vi "HAND_AUTO.vi"() -> ()   [LabVIEW 2014]
uses:
  <vilib>/Platform/TimedLoop/XDataNode/timing_clust.ctl
  <vilib>/Platform/TimedLoop/XDataNode/nitl_modes.ctl
  <vilib>/Platform/TimedLoop/XDataNode/wakeup.ctl
  <vilib>/platform/TimedLoop/XDataNode/XDataNode.xnode
  <vilib>/Platform/TimedLoop/XDataNode/XDNodeRunTimeDep.lvlib
panel:
  out "EMERGENCY":bool
  out "TIME":bool
  out "HAND/AUTO":bool
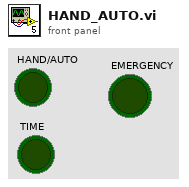
[diagram p1: front panel]
types:
  T1 = typedef "XDNodeRunTimeDep.lvlib/timing_clust.ctl" = cluster{"Expected End [f-1]":u64, "Actual End [f-1]":u64, "Finished Late? [f-1]":bool, "Expected End [i-1]":u64, "Actual End [i-1]":u64, "Finished Late? [i-1]":bool, "Expected Start [i]":u64, "Actual Start [i]":u64, "Expected Start [f]":u64, "Actual Start [f]":u64, "Source Name":string, "Structure Name":string, "Period":i64, "Deadline":i64, "Offset":i64, "Start":i64, "Priority":i32, "Timeout":i32, "Mode":T2, "Wakeup Reason":T3, "Error":errorcluster, "Source Type":string, "Secondary Source Type":string, "Global End Time":u64, "Global Start Time":u64, "Frame Duration":u64, "Iteration Duration":u64, "Assigned CPU":i32, "I/O Scan Engine Mode":u32}
  T2 = typedef "XDNodeRunTimeDep.lvlib/nitl_modes.ctl" = enum32{"No Change", "Process missed periods, maintain original phase", "Discard missed periods, maintain original phase", "Process missed periods, ignore original phase", "Discard missed periods, ignore original phase"}
  T3 = typedef "XDNodeRunTimeDep.lvlib/wakeup.ctl" = enum32{"Normal", "Aborted", "Asynchronous wakeup", "Timing source error", "Timed loop error", "Timeout"}
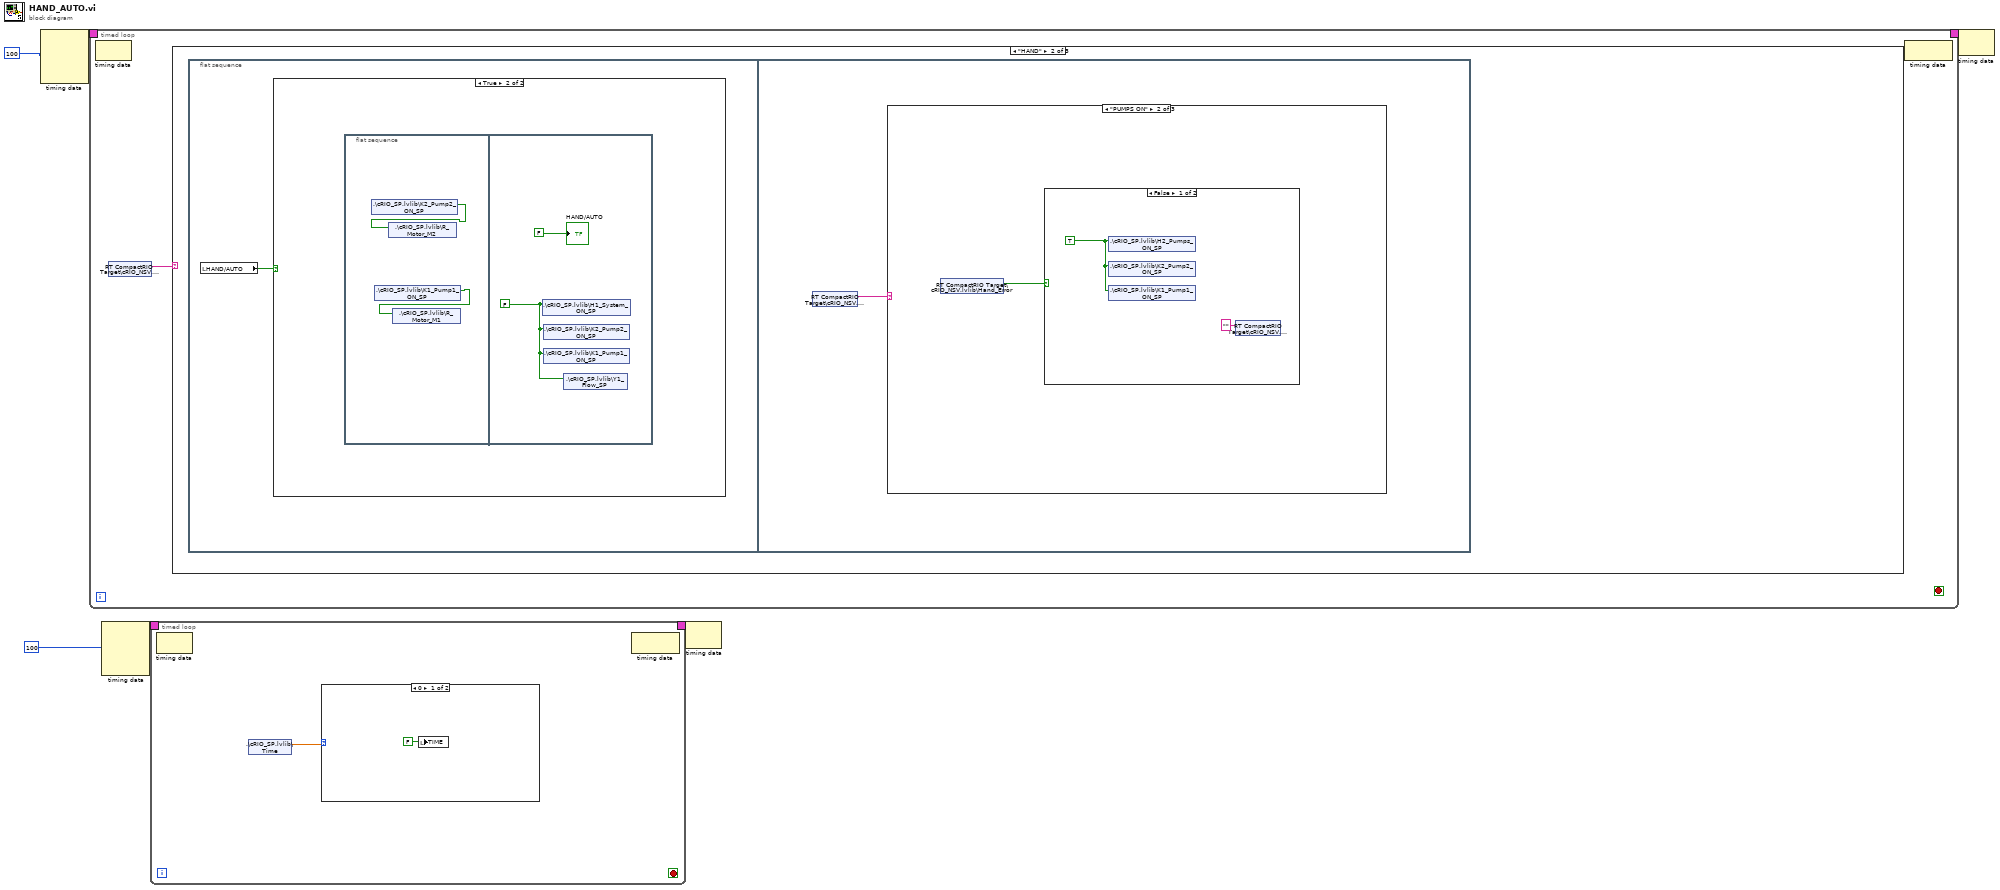
[diagram p0: block diagram]
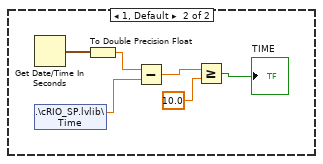
[diagram p2: hidden frame]
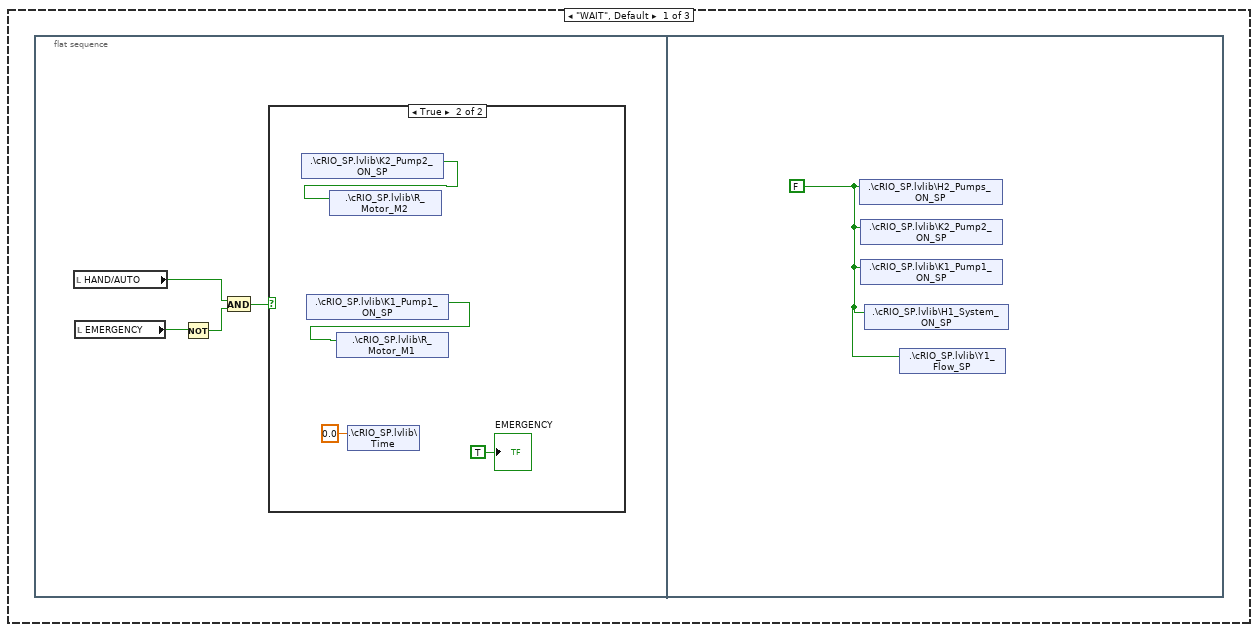
[diagram p3: hidden frame]
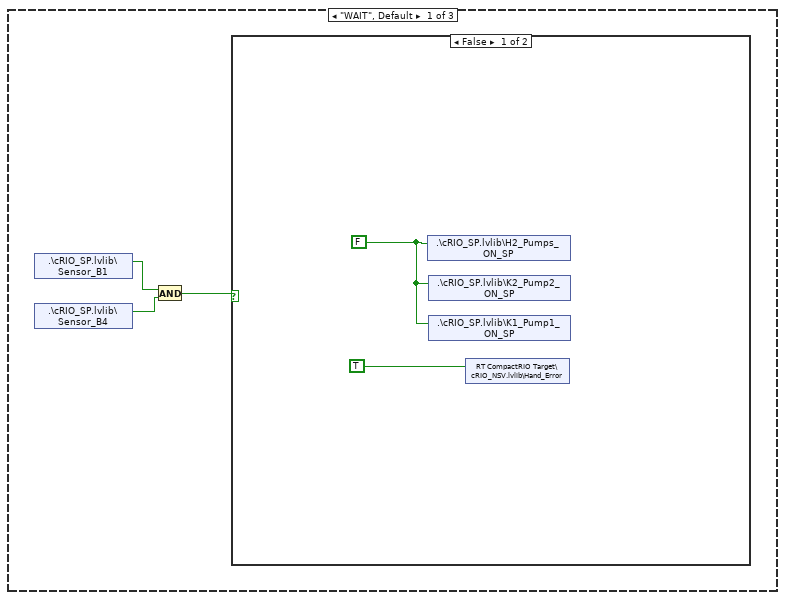
[diagram p6: hidden frame]
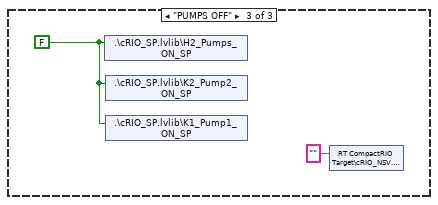
[diagram p9: hidden frame]
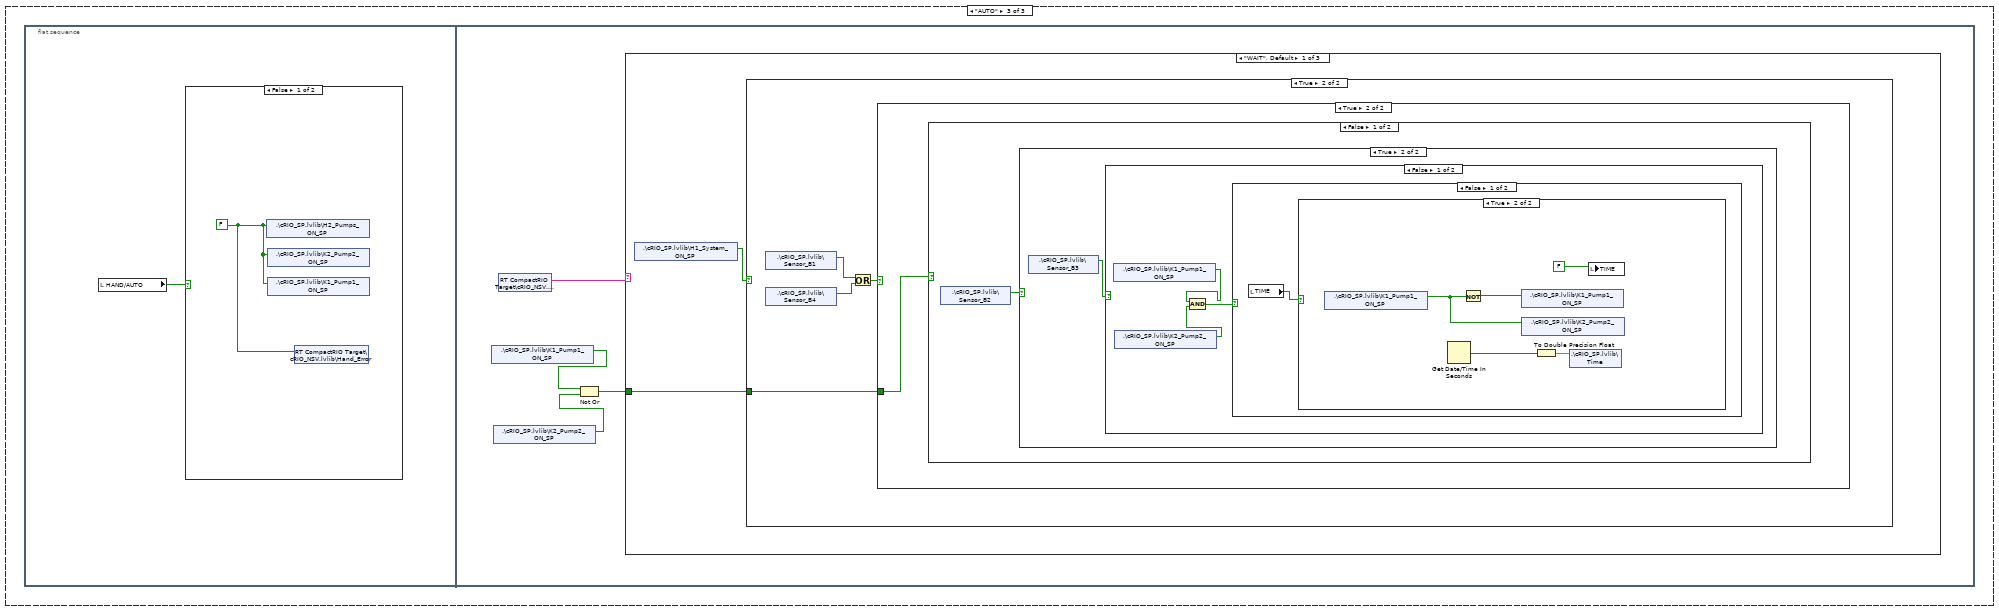
[diagram p10: hidden frame]
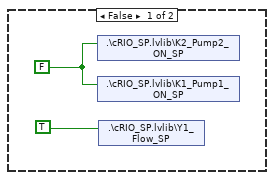
[diagram p13: hidden frame]
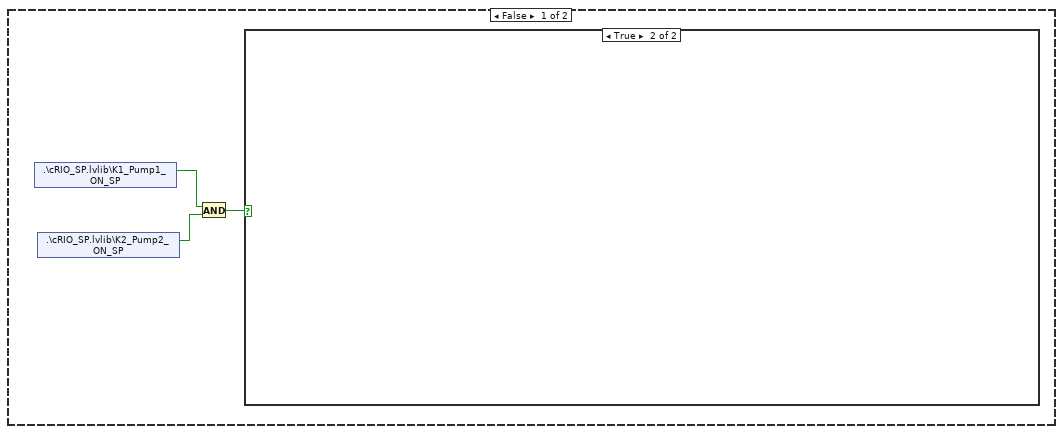
[diagram p14: hidden frame]
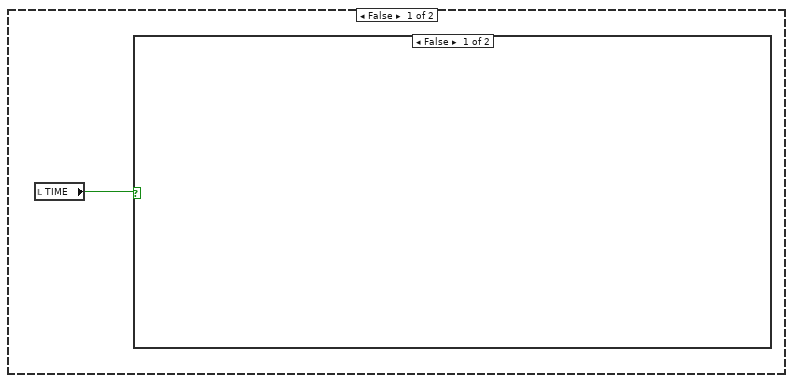
[diagram p15: hidden frame]
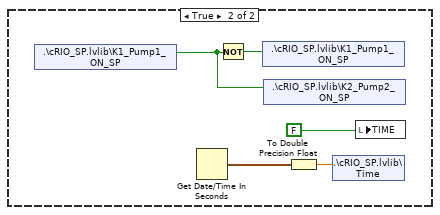
[diagram p16: hidden frame]
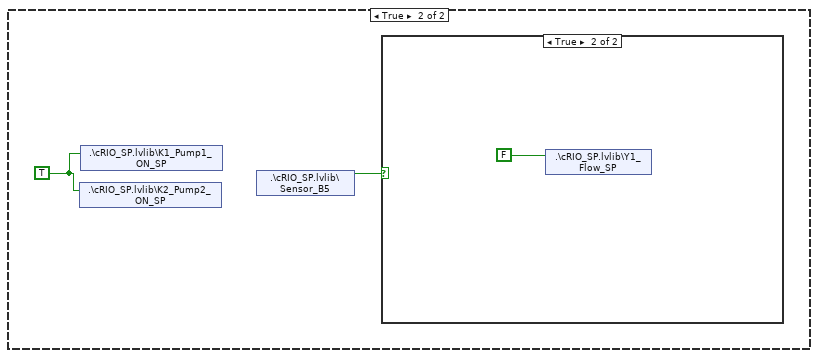
[diagram p19: hidden frame]
diagram:
  n1 = node-c288(i64 100 ("Period")) -> (w6:T1)  [unwired: 3 in]
  n2 = timed-loop {
    timing: w6 -> [_]
    timing-out: [_] -> w5
    stop <- _ stop-if-true
    n3 = node-c288() -> ()  [unwired: 1 in, 1 out]
    n4 = shared-variable "RT CompactRIO Target\\cRIO_NSV.lvlib\\State"() -> (w7:string)  [unwired: 1 in, 1 out]
    n5 = case shown="\"HAND\"" w7 {
      frame "WAIT", Default {
        n6 = flat-sequence {
          frame #0 {
            n7 = local read "HAND/AUTO"() -> (w10:bool)
            n8 = local read "EMERGENCY"() -> (w12:bool)
            n9 = Not(x=w12) -> (.not. x?=w11:bool)
            n10 = And(x=w10, y=w11) -> (x .and. y?=w13:bool)
            n11 = case shown="True" w13 {
              frame False {
              }
              frame True {
                n12 = shared-variable ".\\cRIO_SP.lvlib\\K2_Pump2_ON_SP"() -> (w17:bool)  [unwired: 1 in, 1 out]
                n13 = shared-variable ".\\cRIO_SP.lvlib\\K1_Pump1_ON_SP"() -> (w16:bool)  [unwired: 1 in, 1 out]
                n14 = shared-variable ".\\cRIO_SP.lvlib\\R_Motor_M2"(w17) -> ()  [unwired: 1 in, 1 out]
                n15 = shared-variable ".\\cRIO_SP.lvlib\\R_Motor_M1"(w16) -> ()  [unwired: 1 in, 1 out]
                n16 = shared-variable ".\\cRIO_SP.lvlib\\Time"(0.0 ("Time")) -> ()  [unwired: 1 in, 1 out]
                "EMERGENCY" <- TRUE ("EMERGENCY")
              }
            }
          }
          frame #1 {
            w18 = FALSE
            n17 = shared-variable ".\\cRIO_SP.lvlib\\H2_Pumps_ON_SP"(w18) -> ()  [unwired: 1 in, 1 out]
            n18 = shared-variable ".\\cRIO_SP.lvlib\\K2_Pump2_ON_SP"(w18) -> ()  [unwired: 1 in, 1 out]
            n19 = shared-variable ".\\cRIO_SP.lvlib\\K1_Pump1_ON_SP"(w18) -> ()  [unwired: 1 in, 1 out]
            n20 = shared-variable ".\\cRIO_SP.lvlib\\H1_System_ON_SP"(w18) -> ()  [unwired: 1 in, 1 out]
            n21 = shared-variable ".\\cRIO_SP.lvlib\\Y1_Flow_SP"(w18) -> ()  [unwired: 1 in, 1 out]
          }
        }
      }
      frame "HAND" {
        n22 = flat-sequence {
          frame #0 {
            n23 = local read "HAND/AUTO"() -> (w19:bool)
            n24 = case shown="True" w19 {
              frame False {
              }
              frame True {
                n25 = flat-sequence {
                  frame #0 {
                    n26 = shared-variable ".\\cRIO_SP.lvlib\\K2_Pump2_ON_SP"() -> (w20:bool)  [unwired: 1 in, 1 out]
                    n27 = shared-variable ".\\cRIO_SP.lvlib\\K1_Pump1_ON_SP"() -> (w21:bool)  [unwired: 1 in, 1 out]
                    n28 = shared-variable ".\\cRIO_SP.lvlib\\R_Motor_M2"(w20) -> ()  [unwired: 1 in, 1 out]
                    n29 = shared-variable ".\\cRIO_SP.lvlib\\R_Motor_M1"(w21) -> ()  [unwired: 1 in, 1 out]
                  }
                  frame #1 {
                    w23 = FALSE
                    n30 = shared-variable ".\\cRIO_SP.lvlib\\H1_System_ON_SP"(w23) -> ()  [unwired: 1 in, 1 out]
                    n31 = shared-variable ".\\cRIO_SP.lvlib\\K2_Pump2_ON_SP"(w23) -> ()  [unwired: 1 in, 1 out]
                    n32 = shared-variable ".\\cRIO_SP.lvlib\\K1_Pump1_ON_SP"(w23) -> ()  [unwired: 1 in, 1 out]
                    n33 = shared-variable ".\\cRIO_SP.lvlib\\Y1_Flow_SP"(w23) -> ()  [unwired: 1 in, 1 out]
                    "HAND/AUTO" <- FALSE
                  }
                }
              }
            }
          }
          frame #1 {
            n34 = shared-variable "RT CompactRIO Target\\cRIO_NSV.lvlib\\Tasks"() -> (w24:string)  [unwired: 1 in, 1 out]
            n35 = case shown="\"PUMPS ON\"" w24 {
              frame "WAIT", Default {
                n36 = shared-variable ".\\cRIO_SP.lvlib\\Sensor_B1"() -> (w26:bool)  [unwired: 1 in, 1 out]
                n37 = shared-variable ".\\cRIO_SP.lvlib\\Sensor_B4"() -> (w27:bool)  [unwired: 1 in, 1 out]
                n38 = And(x=w26, y=w27) -> (x .and. y?=w25:bool)
                n39 = case shown="False" w25 {
                  frame False {
                    w29 = FALSE
                    n40 = shared-variable ".\\cRIO_SP.lvlib\\H2_Pumps_ON_SP"(w29) -> ()  [unwired: 1 in, 1 out]
                    n41 = shared-variable ".\\cRIO_SP.lvlib\\K2_Pump2_ON_SP"(w29) -> ()  [unwired: 1 in, 1 out]
                    n42 = shared-variable ".\\cRIO_SP.lvlib\\K1_Pump1_ON_SP"(w29) -> ()  [unwired: 1 in, 1 out]
                    n43 = shared-variable "RT CompactRIO Target\\cRIO_NSV.lvlib\\Hand_Error"(TRUE) -> ()  [unwired: 1 in, 1 out]
                  }
                  frame True {
                  }
                }
              }
              frame "PUMPS ON" {
                n44 = shared-variable "RT CompactRIO Target\\cRIO_NSV.lvlib\\Hand_Error"() -> (w30:bool)  [unwired: 1 in, 1 out]
                n45 = case shown="False" w30 {
                  frame False {
                    w32 = TRUE
                    n46 = shared-variable ".\\cRIO_SP.lvlib\\H2_Pumps_ON_SP"(w32) -> ()  [unwired: 1 in, 1 out]
                    n47 = shared-variable ".\\cRIO_SP.lvlib\\K2_Pump2_ON_SP"(w32) -> ()  [unwired: 1 in, 1 out]
                    n48 = shared-variable ".\\cRIO_SP.lvlib\\K1_Pump1_ON_SP"(w32) -> ()  [unwired: 1 in, 1 out]
                    n49 = shared-variable "RT CompactRIO Target\\cRIO_NSV.lvlib\\Tasks"("" ("Tasks")) -> ()  [unwired: 1 in, 1 out]
                  }
                  frame True {
                  }
                }
              }
              frame "PUMPS OFF" {
                w34 = FALSE
                n50 = shared-variable ".\\cRIO_SP.lvlib\\H2_Pumps_ON_SP"(w34) -> ()  [unwired: 1 in, 1 out]
                n51 = shared-variable ".\\cRIO_SP.lvlib\\K2_Pump2_ON_SP"(w34) -> ()  [unwired: 1 in, 1 out]
                n52 = shared-variable ".\\cRIO_SP.lvlib\\K1_Pump1_ON_SP"(w34) -> ()  [unwired: 1 in, 1 out]
                n53 = shared-variable "RT CompactRIO Target\\cRIO_NSV.lvlib\\Tasks"("" ("Tasks")) -> ()  [unwired: 1 in, 1 out]
              }
            }
          }
        }
      }
      frame "AUTO" {
        n54 = flat-sequence {
          frame #0 {
            n55 = local read "HAND/AUTO"() -> (w35:bool)
            n56 = case shown="False" w35 {
              frame False {
                w36 = FALSE
                n57 = shared-variable ".\\cRIO_SP.lvlib\\H2_Pumps_ON_SP"(w36) -> ()  [unwired: 1 in, 1 out]
                n58 = shared-variable ".\\cRIO_SP.lvlib\\K2_Pump2_ON_SP"(w36) -> ()  [unwired: 1 in, 1 out]
                n59 = shared-variable ".\\cRIO_SP.lvlib\\K1_Pump1_ON_SP"(w36) -> ()  [unwired: 1 in, 1 out]
                n60 = shared-variable "RT CompactRIO Target\\cRIO_NSV.lvlib\\Hand_Error"(w36) -> ()  [unwired: 1 in, 1 out]
              }
              frame True {
              }
            }
          }
          frame #1 {
            n61 = shared-variable ".\\cRIO_SP.lvlib\\K1_Pump1_ON_SP"() -> (w38:bool)  [unwired: 1 in, 1 out]
            n62 = shared-variable ".\\cRIO_SP.lvlib\\K2_Pump2_ON_SP"() -> (w37:bool)  [unwired: 1 in, 1 out]
            n63 = shared-variable "RT CompactRIO Target\\cRIO_NSV.lvlib\\Tasks"() -> (w40:string)  [unwired: 1 in, 1 out]
            n64 = Not Or(1:w37, 2:w38) -> (0:w39:bool)
            n65 = case shown="\"WAIT\", Default" w40 {
              tunnel: w39 -> [w41 _ _]
              frame "WAIT", Default {
                n66 = shared-variable ".\\cRIO_SP.lvlib\\H1_System_ON_SP"() -> (w42:bool)  [unwired: 1 in, 1 out]
                n67 = case shown="True" w42 {
                  tunnel: w41 -> [_ w44]
                  frame False {
                  }
                  frame True {
                    n68 = shared-variable ".\\cRIO_SP.lvlib\\Sensor_B1"() -> (w43:bool)  [unwired: 1 in, 1 out]
                    n69 = shared-variable ".\\cRIO_SP.lvlib\\Sensor_B4"() -> (w45:bool)  [unwired: 1 in, 1 out]
                    n70 = Or(x=w43, y=w45) -> (x .or. y?=w46:bool)
                    n71 = case shown="True" w46 {
                      tunnel: w44 -> [_ w49]
                      frame False {
                        w48 = FALSE
                        n72 = shared-variable ".\\cRIO_SP.lvlib\\K2_Pump2_ON_SP"(w48) -> ()  [unwired: 1 in, 1 out]
                        n73 = shared-variable ".\\cRIO_SP.lvlib\\K1_Pump1_ON_SP"(w48) -> ()  [unwired: 1 in, 1 out]
                        n74 = shared-variable ".\\cRIO_SP.lvlib\\Y1_Flow_SP"(TRUE) -> ()  [unwired: 1 in, 1 out]
                      }
                      frame True {
                        n75 = case shown="False" w49 {
                          frame False {
                            n76 = shared-variable ".\\cRIO_SP.lvlib\\Sensor_B2"() -> (w50:bool)  [unwired: 1 in, 1 out]
                            n77 = case shown="True" w50 {
                              frame False {
                                n78 = shared-variable ".\\cRIO_SP.lvlib\\K1_Pump1_ON_SP"() -> (w51:bool)  [unwired: 1 in, 1 out]
                                n79 = shared-variable ".\\cRIO_SP.lvlib\\K2_Pump2_ON_SP"() -> (w52:bool)  [unwired: 1 in, 1 out]
                                n80 = And(x=w51, y=w52) -> (x .and. y?=w53:bool)
                                n81 = case shown="True" w53 {
                                frame False {
                                n82 = local read "TIME"() -> (w54:bool)
                                n83 = case shown="False" w54 {
                                frame False {
                                }
                                frame True {
                                n84 = shared-variable ".\\cRIO_SP.lvlib\\K1_Pump1_ON_SP"() -> (w58:bool)  [unwired: 1 in, 1 out]
                                n85 = Get Date/Time In Seconds() -> (seconds since 1Jan1904=w55:timestamp)
                                n86 = Not(x=w58) -> (.not. x?=w59:bool)
                                n87 = shared-variable ".\\cRIO_SP.lvlib\\K1_Pump1_ON_SP"(w59) -> ()  [unwired: 1 in, 1 out]
                                n88 = shared-variable ".\\cRIO_SP.lvlib\\K2_Pump2_ON_SP"(w58) -> ()  [unwired: 1 in, 1 out]
                                n89 = To Double Precision Float(number=w55) -> (double precision float=w56:dbl)
                                n90 = shared-variable ".\\cRIO_SP.lvlib\\Time"(w56) -> ()  [unwired: 1 in, 1 out]
                                n91 = local write "TIME"(FALSE) -> ()
                                }
                                }
                                }
                                frame True {
                                }
                                }
                              }
                              frame True {
                                n92 = shared-variable ".\\cRIO_SP.lvlib\\Sensor_B3"() -> (w60:bool)  [unwired: 1 in, 1 out]
                                n93 = case shown="False" w60 {
                                frame False {
                                n94 = shared-variable ".\\cRIO_SP.lvlib\\K1_Pump1_ON_SP"() -> (w62:bool)  [unwired: 1 in, 1 out]
                                n95 = shared-variable ".\\cRIO_SP.lvlib\\K2_Pump2_ON_SP"() -> (w61:bool)  [unwired: 1 in, 1 out]
                                n96 = And(x=w62, y=w61) -> (x .and. y?=w63:bool)
                                n97 = case shown="False" w63 {
                                frame False {
                                n98 = local read "TIME"() -> (w64:bool)
                                n99 = case shown="True" w64 {
                                frame False {
                                }
                                frame True {
                                n100 = shared-variable ".\\cRIO_SP.lvlib\\K1_Pump1_ON_SP"() -> (w68:bool)  [unwired: 1 in, 1 out]
                                n101 = Get Date/Time In Seconds() -> (seconds since 1Jan1904=w65:timestamp)
                                n102 = Not(x=w68) -> (.not. x?=w69:bool)
                                n103 = shared-variable ".\\cRIO_SP.lvlib\\K1_Pump1_ON_SP"(w69) -> ()  [unwired: 1 in, 1 out]
                                n104 = shared-variable ".\\cRIO_SP.lvlib\\K2_Pump2_ON_SP"(w68) -> ()  [unwired: 1 in, 1 out]
                                n105 = To Double Precision Float(number=w65) -> (double precision float=w66:dbl)
                                n106 = shared-variable ".\\cRIO_SP.lvlib\\Time"(w66) -> ()  [unwired: 1 in, 1 out]
                                n107 = local write "TIME"(FALSE) -> ()
                                }
                                }
                                }
                                frame True {
                                }
                                }
                                }
                                frame True {
                                w71 = TRUE
                                n108 = shared-variable ".\\cRIO_SP.lvlib\\K2_Pump2_ON_SP"(w71) -> ()  [unwired: 1 in, 1 out]
                                n109 = shared-variable ".\\cRIO_SP.lvlib\\K1_Pump1_ON_SP"(w71) -> ()  [unwired: 1 in, 1 out]
                                n110 = shared-variable ".\\cRIO_SP.lvlib\\Sensor_B5"() -> (w70:bool)  [unwired: 1 in, 1 out]
                                n111 = case shown="True" w70 {
                                frame False {
                                }
                                frame True {
                                n112 = shared-variable ".\\cRIO_SP.lvlib\\Y1_Flow_SP"(FALSE) -> ()  [unwired: 1 in, 1 out]
                                }
                                }
                                }
                                }
                              }
                            }
                          }
                          frame True {
                            n113 = shared-variable ".\\cRIO_SP.lvlib\\Sensor_B2"() -> (w73:bool)  [unwired: 1 in, 1 out]
                            n114 = case shown="True" w73 {
                              frame False {
                              }
                              frame True {
                                n115 = Get Date/Time In Seconds() -> (seconds since 1Jan1904=w74:timestamp)
                                n116 = shared-variable ".\\cRIO_SP.lvlib\\K1_Pump1_ON_SP"(TRUE) -> ()  [unwired: 1 in, 1 out]
                                n117 = To Double Precision Float(number=w74) -> (double precision float=w75:dbl)
                                n118 = shared-variable ".\\cRIO_SP.lvlib\\Time"(w75) -> ()  [unwired: 1 in, 1 out]
                              }
                            }
                          }
                        }
                      }
                    }
                  }
                }
              }
              frame "SYSTEM ON" {
                w80 = TRUE
                n119 = shared-variable ".\\cRIO_SP.lvlib\\R_Motor_M1"() -> (w78:bool)  [unwired: 1 in, 1 out]
                n120 = shared-variable ".\\cRIO_SP.lvlib\\R_Motor_M2"() -> (w77:bool)  [unwired: 1 in, 1 out]
                n121 = shared-variable ".\\cRIO_SP.lvlib\\Y1_Flow_SP"(w80) -> ()  [unwired: 1 in, 1 out]
                n122 = shared-variable ".\\cRIO_SP.lvlib\\H1_System_ON_SP"(w80) -> ()  [unwired: 1 in, 1 out]
                n123 = shared-variable ".\\cRIO_SP.lvlib\\K1_Pump1_ON_SP"(w78) -> ()  [unwired: 1 in, 1 out]
                n124 = shared-variable ".\\cRIO_SP.lvlib\\K2_Pump2_ON_SP"(w77) -> ()  [unwired: 1 in, 1 out]
                n125 = shared-variable "RT CompactRIO Target\\cRIO_NSV.lvlib\\Tasks"("" ("Tasks")) -> ()  [unwired: 1 in, 1 out]
              }
              frame "SYSTEM OFF" {
                n126 = flat-sequence {
                  frame #0 {
                    n127 = local read "HAND/AUTO"() -> (w82:bool)
                    n128 = local read "EMERGENCY"() -> (w84:bool)
                    n129 = Not(x=w84) -> (.not. x?=w81:bool)
                    n130 = And(x=w82, y=w81) -> (x .and. y?=w83:bool)
                    n131 = case shown="True" w83 {
                      frame False {
                        n132 = Get Date/Time In Seconds() -> (seconds since 1Jan1904=w85:timestamp)
                        n133 = To Double Precision Float(number=w85) -> (double precision float=w86:dbl)
                        n134 = local write "HAND/AUTO"(TRUE) -> ()
                        n135 = local write "EMERGENCY"(FALSE) -> ()
                        n136 = shared-variable ".\\cRIO_SP.lvlib\\Time"(w86) -> ()  [unwired: 1 in, 1 out]
                      }
                      frame True {
                        n137 = shared-variable ".\\cRIO_SP.lvlib\\K1_Pump1_ON_SP"() -> (w89:bool)  [unwired: 1 in, 1 out]
                        n138 = shared-variable ".\\cRIO_SP.lvlib\\K2_Pump2_ON_SP"() -> (w90:bool)  [unwired: 1 in, 1 out]
                        n139 = shared-variable ".\\cRIO_SP.lvlib\\R_Motor_M1"(w89) -> ()  [unwired: 1 in, 1 out]
                        n140 = shared-variable ".\\cRIO_SP.lvlib\\R_Motor_M2"(w90) -> ()  [unwired: 1 in, 1 out]
                      }
                    }
                  }
                  frame #1 {
                    w91 = FALSE
                    n141 = shared-variable ".\\cRIO_SP.lvlib\\Y1_Flow_SP"(w91) -> ()  [unwired: 1 in, 1 out]
                    n142 = shared-variable ".\\cRIO_SP.lvlib\\H1_System_ON_SP"(w91) -> ()  [unwired: 1 in, 1 out]
                    n143 = shared-variable ".\\cRIO_SP.lvlib\\K1_Pump1_ON_SP"(w91) -> ()  [unwired: 1 in, 1 out]
                    n144 = shared-variable ".\\cRIO_SP.lvlib\\K2_Pump2_ON_SP"(w91) -> ()  [unwired: 1 in, 1 out]
                    n145 = shared-variable "RT CompactRIO Target\\cRIO_NSV.lvlib\\Tasks"("" ("Tasks")) -> ()  [unwired: 1 in, 1 out]
                  }
                }
              }
            }
          }
        }
      }
    }
    n146 = node-c288() -> ()  [unwired: 1 in, 1 out]
  }
  n147 = node-c288(i64 100 ("Period")) -> (w3:T1)  [unwired: 3 in]
  n148 = timed-loop {
    timing: w3 -> [_]
    timing-out: [_] -> w2
    stop <- _ stop-if-true
    n149 = node-c288() -> ()  [unwired: 1 in, 1 out]
    n150 = shared-variable ".\\cRIO_SP.lvlib\\Time"() -> (w93:dbl)  [unwired: 1 in, 1 out]
    n151 = case shown="0" w93 {
      frame 0 {
        n152 = local write "TIME"(FALSE ("TIME")) -> ()
      }
      frame 1, Default {
        n153 = Get Date/Time In Seconds() -> (seconds since 1Jan1904=w100:timestamp)
        n154 = shared-variable ".\\cRIO_SP.lvlib\\Time"() -> (w96:dbl)  [unwired: 1 in, 1 out]
        n155 = To Double Precision Float(number=w100) -> (double precision float=w97:dbl)
        n156 = Subtract(x=w97, y=w96) -> (x-y=w98:dbl)
        n157 = Greater Or Equal?(x=w98, y=10.0) -> (x >= y?=→"TIME":bool)
      }
    }
    n158 = node-c288() -> ()  [unwired: 1 in, 1 out]
  }
  n159 = node-c288(w2) -> ()  [unwired: 1 out]
  n160 = node-c288(w5) -> ()  [unwired: 1 out]
